vi "RANDOMGENERATOR.vi"() -> (1 "Boolean 4":bool, 2 "Boolean 2":bool, 3 "Boolean 3":bool, 4 "index of element":i32, 5 "Boolean":bool)   [LabVIEW 2021]
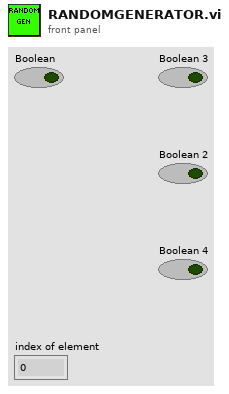
[diagram p1: front panel]
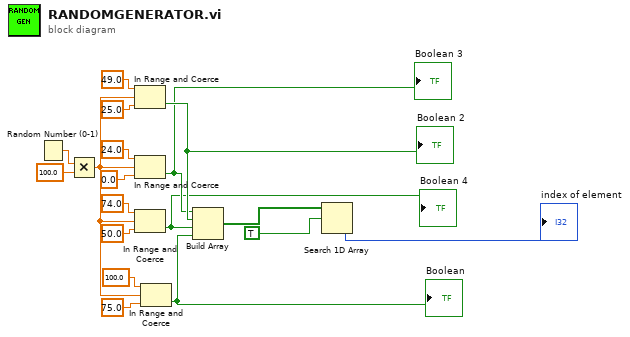
[diagram p0: block diagram]
diagram:
  n1 = Random Number (0-1)() -> (number: 0 to 1=w1:dbl)
  n2 = Multiply(x=w1, y=100.0) -> (x*y=w2:dbl)
  n3 = In Range and Coerce(upper limit=49.0, x=w2, lower limit=25.0) -> (In Range?=w16:bool)  [unwired: 1 out]
  "Boolean 2" <- w16
  n4 = In Range and Coerce(upper limit=24.0, x=w2, lower limit=0.0) -> (In Range?=w15:bool)  [unwired: 1 out]
  "Boolean 3" <- w15
  n5 = In Range and Coerce(upper limit=74.0, x=w2, lower limit=50.0) -> (In Range?=w14:bool)  [unwired: 1 out]
  "Boolean 4" <- w14
  n6 = In Range and Coerce(upper limit=100.0, x=w2, lower limit=75.0) -> (In Range?=w17:bool)  [unwired: 1 out]
  "Boolean" <- w17
  n7 = Build Array(w15, w16, w14, w17) -> (w3:bool[])
  n8 = Search 1D Array(1D array=w3, element=TRUE) -> (index of element=→"index of element":i32)  [unwired: 1 in]
